vi "LoadComplexArrayFromFile.vi"(8 "error in":errorcluster, 11 "SourceFileName":string) -> (0 "error out":errorcluster, 3 "Array":csg[](array[numeric]))   [LabVIEW 2015]
panel:
  out "appended path":path
  out "Application Directory":path
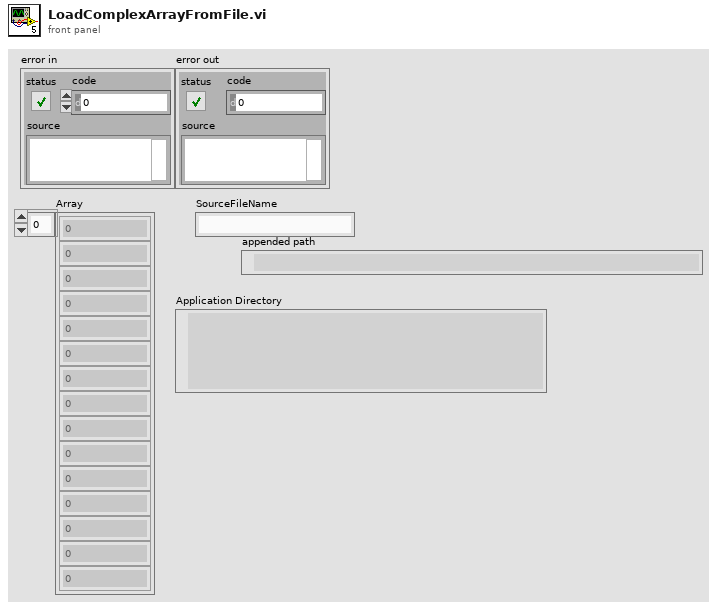
[diagram p1: front panel]
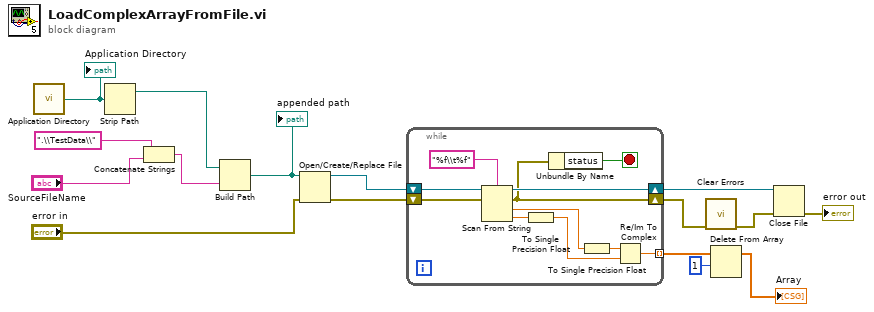
[diagram p0: block diagram]
diagram:
  n1 = call <vilib>:"Application Directory.vi"() -> ("Application Directory"=w10:path)
  "Application Directory" <- w10
  n2 = Strip Path(path=w10) -> (stripped path=w4:path)  [unwired: 1 out]
  n3 = Concatenate Strings(".\\TestData\\" ("string"), "SourceFileName") -> (w3:string)
  n4 = Build Path(base path=w4, name or relative path=w3) -> (appended path=w9:path)
  "appended path" <- w9
  n5 = Open/Create/Replace File(file path (use dialog)=w9, error in="error in") -> (refnum out=w15:refnum<file>, error out=w14:errorcluster)  [unwired: 4 in, 1 out]
  n6 = while {
    shift-right: [w24] -> w12
    shift-left: w15 -> [w27]
    shift-right: [w20] -> w13
    shift-left: w14 -> [w26]
    tunnel: [w21] -> w8 mode=indexing
    stop <- w19 stop-if-true
    n7 = Scan From String("%f\\t%f" ("format string"), w27, w26) -> (w24:refnum<file>, w20:errorcluster, output 1=w23:dbl, output 2=w22:dbl)  [unwired: 2 in]
    n8 = To Single Precision Float(number=w22) -> (single precision float=w18:sgl)
    n9 = Unbundle By Name(w20) -> ("status"=w19:bool)
    n10 = To Single Precision Float(number=w23) -> (single precision float=w17:sgl)
    n11 = Re/Im To Complex(1:w18, 2:w17) -> (0:w21:csg)
  }
  n12 = call <vilib>:"Clear Errors.vi"("error in (no error)"=w13) -> ("error out"=w5:errorcluster)  [unwired: 5 in, 1 out]
  n13 = Delete From Array(array=w8, length=1) -> (array with subset deleted=→"Array":csg[])  [unwired: 1 in, 1 out]
  n14 = Close File(refnum=w12, error in=w5) -> (error out=→"error out":errorcluster)  [unwired: 1 out]
